vi "adam-4069-channel.vi"() -> ()   [LabVIEW 2024]
panel:
  in  "baud rate (19200)":u32=19200
  in  "COM Port (COM10)":refnum<visa-resource-name>="COM10"
  in  "Stop Program":bool
  in  "Stop All":bool
  out "Status":string
  out "command":string
  in  "Channel Number":dbl=1.0 min=1.0 max=9.0 step=1.0
  in  "Channel Active":bool
  out "read buffer":string
  out "Bytes Written":u32
  out "Channel Active":bool
  out "error out":errorcluster
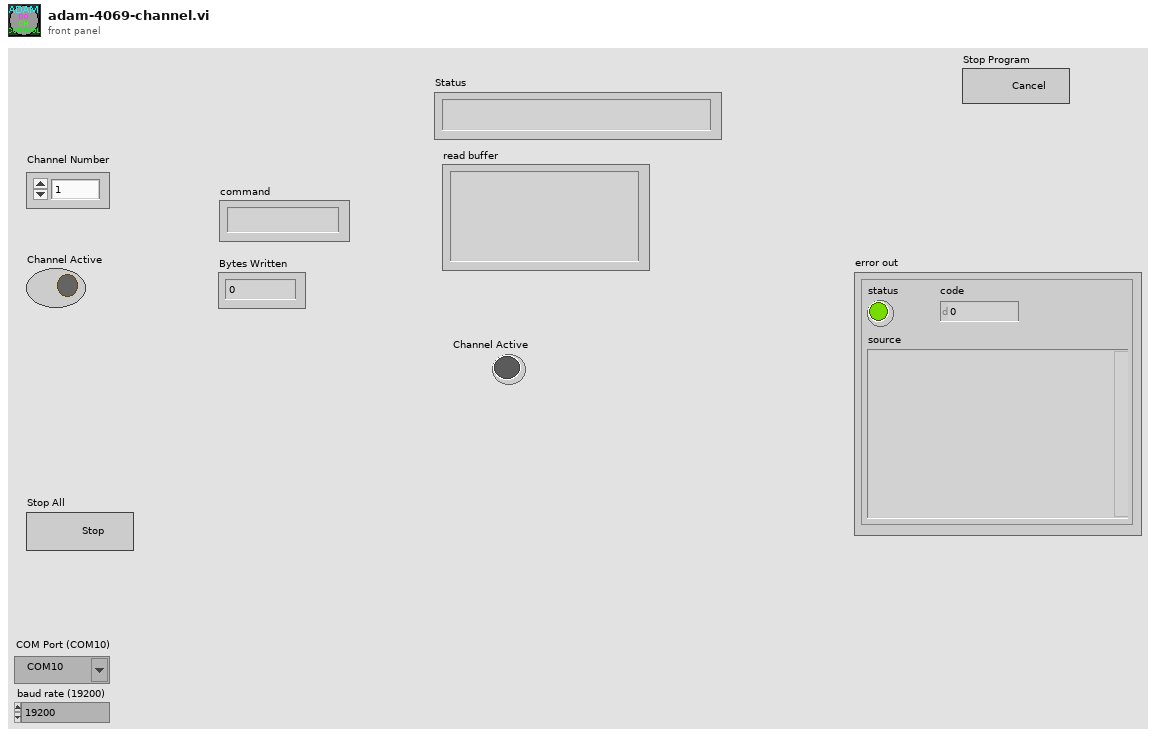
[diagram p1: front panel]
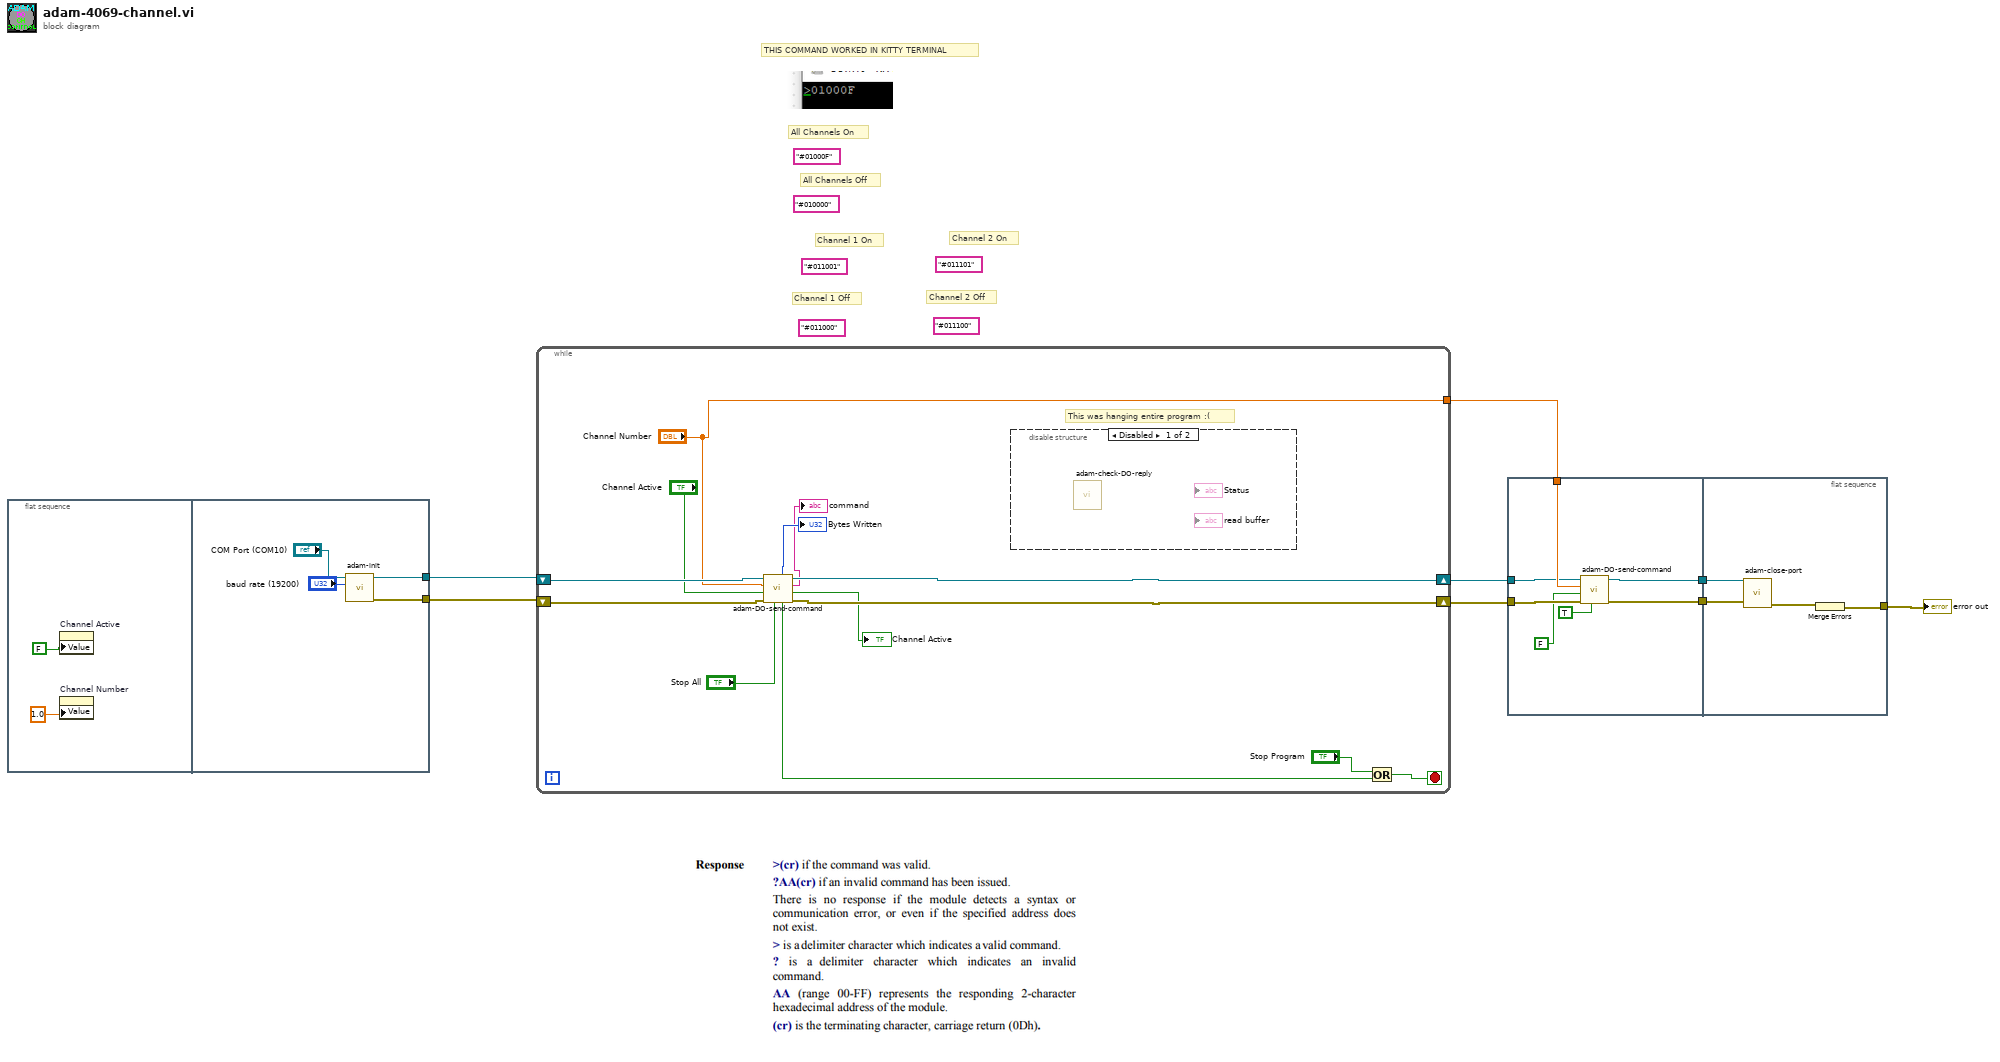
[diagram p0: block diagram]
diagram:
  (unwired) "#011101" ("write buffer")
  (unwired) "#011100" ("write buffer")
  (unwired) "#011001" ("write buffer")
  (unwired) "#011000" ("write buffer")
  (unwired) "#010000" ("write buffer")
  (unwired) "#01000F" ("write buffer")
  # "Channel 2 Off"
  # "Channel 2 On"
  # "Channel 1 Off"
  # "Channel 1 On"
  # "All Channels Off"
  # "All Channels On"
  # "THIS COMMAND WORKED IN KITTY TERMINAL"
  n1 = flat-sequence {
    tunnel: [w14] -> w5
    tunnel: [w13] -> w4
    frame #0 {
      n2 = property on="Channel Active" class="Bool (strict)"("Value"=FALSE ("Channel Active")) -> ()  [unwired: 2 in, 2 out]
      n3 = property on="Channel Number" class="DigNum (strict)"("Value"=1.0 ("Channel Number")) -> ()  [unwired: 2 in, 2 out]
    }
    frame #1 {
      n4 = call "adam-init.vi"("baud rate (19200)"="baud rate (19200)", "COM Port (COM10)"="COM Port (COM10)") -> ("error out"=w13:errorcluster, "VISA resource name out"=w14:refnum<visa-resource-name>)  [unwired: 8 in]
    }
  }
  n5 = while {
    shift-right: [w18] -> w6
    shift-left: w5 -> [w27]
    shift-right: [w17] -> w8
    shift-left: w4 -> [w26]
    tunnel: ["Channel Number"] -> w7
    stop <- w21 stop-if-true
    # "This was hanging entire program :("
    n6 = call "adam-DO-send-command.vi"("Stop All"="Stop All", "error in (no error)"=w26, "Channel Active"="Channel Active", "Channel Number"="Channel Number", "VISA Refnum in"=w27) -> ("error out"=w17:errorcluster, "Desired State"=→"Channel Active":bool, "command"=→"command":string, "VISA Refnum out"=w18:refnum<visa-resource-name>, "STOPPED"=w22:bool, "Bytes Written"=→"Bytes Written":u32)  [unwired: 1 in]
    n7 = disable-structure shown="Disabled" {
      frame Disabled {
        n8 = call "adam-check-DO-reply.vi"() -> ("Channel Active"=w28:bool)  [unwired: 7 in, 4 out]
      }
      frame Enabled {
      }
    }
    n9 = Or(x="Stop Program", y=w22) -> (x .or. y?=w21:bool)
  }
  n10 = flat-sequence {
    tunnel: w8 -> [w35]
    tunnel: w7 -> [w33]
    tunnel: w6 -> [w30]
    tunnel: [w34] -> w3
    tunnel: [w31] -> w2
    tunnel: w3 -> [w37]
    tunnel: w2 -> [w38]
    tunnel: [w36] -> w1
    frame #0 {
      n11 = call "adam-DO-send-command.vi"("Stop All"=TRUE, "error in (no error)"=w35, "Channel Active"=FALSE, "Channel Number"=w33, "VISA Refnum in"=w30) -> ("error out"=w31:errorcluster, "VISA Refnum out"=w34:refnum<visa-resource-name>)  [unwired: 1 in, 4 out]
    }
    frame #1 {
      n12 = call "adam-close-port.vi"("error in (no error)"=w38, "VISA Refnum in"=w37) -> ("error out"=w39:errorcluster)  [unwired: 9 in]
      n13 = Merge Errors(w39) -> (w36:errorcluster)
    }
  }
  "error out" <- w1
